vi "Grow Tail.vi"(8 "Keypress In":enum16{"Right", "Down", "Up", "Left"}(ring), 9 "Map In":u32[][](array[numeric]), 10 "Locations In":cluster{"Location Y":i32, "Location X":i32}[](array[cluster])=[{"Location Y"=12, "Location X"=8}, {"Location Y"=12, "Location X"=7}, {"Location Y"=12, "Location X"=6}, {"Location Y"=12, "Location X"=5}, {"Location Y"=12, "Location X"=4}]) -> (1 "Keypress Out":enum16{"Right", "Down", "Up", "Left"}(ring), 2 "Map Out":u32[][](array[numeric]), 3 "Locations Out":cluster{"Location Y":i32, "Location X":i32}[](array[cluster]))   [LabVIEW 2014]
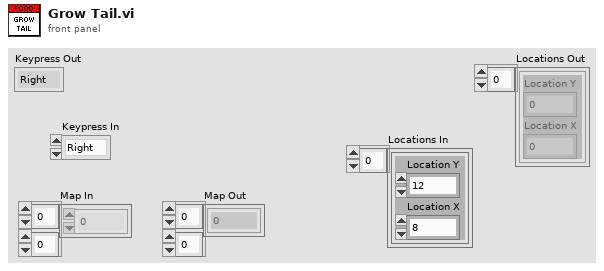
[diagram p1: front panel]
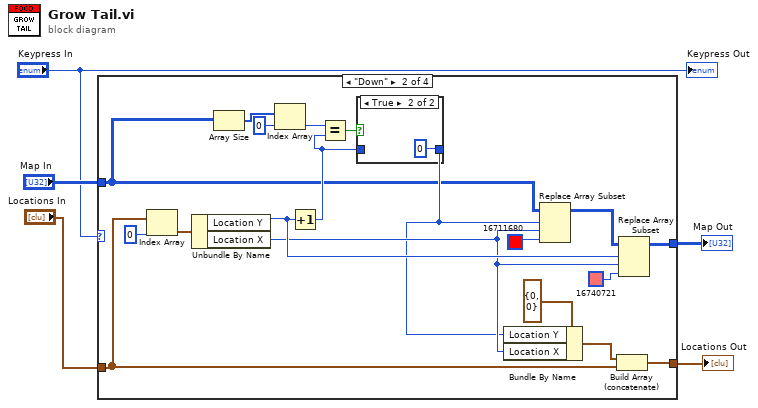
[diagram p0: block diagram]
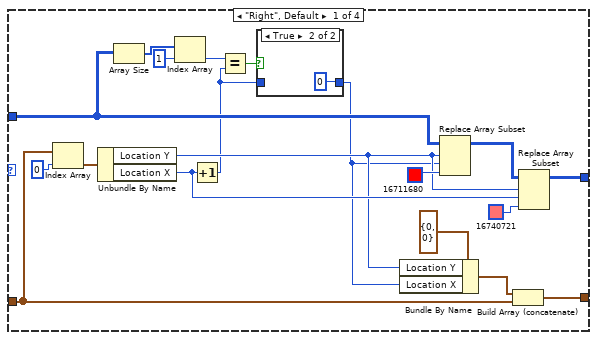
[diagram p2: hidden frame]
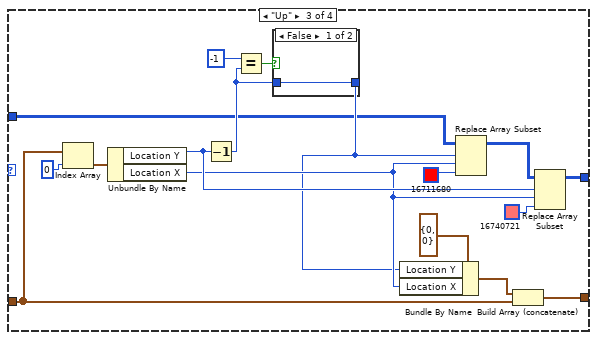
[diagram p5: hidden frame]
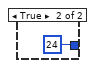
[diagram p6: hidden frame]
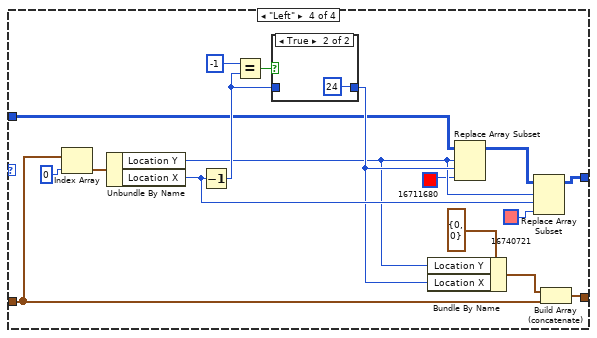
[diagram p7: hidden frame]
diagram:
  n1 = case shown="\"Down\"" "Keypress In" {
    tunnel: [w16 w28 w48 w68] -> w5
    tunnel: "Map In" -> [w13 w30 w51 w69]
    tunnel: [w7 w27 w49 w67] -> w3
    tunnel: "Locations In" -> [w6 w29 w50 w70]
    frame "Right", Default {
      n2 = Index Array(array=w6, index=0) -> (element=w23:cluster{"Location Y":i32, "Location X":i32})
      n3 = Unbundle By Name(w23) -> ("Location Y"=w15:i32, "Location X"=w19:i32)
      n4 = Array Size(array=w13) -> (size(s)=w12:i32[])
      n5 = Index Array(array=w12, index=1) -> (element=w10:i32)
      n6 = Increment(x=w19) -> (x+1=w9:i32)
      n7 = Equal?(x=w10, y=w9) -> (x = y?=w14:bool)
      n8 = case shown="True" w14 {
        tunnel: w9 -> [w25 _]
        tunnel: [w25 0] -> w8
        frame False {
        }
        frame True {
        }
      }
      n9 = Bundle By Name(cluster=cluster{"Location Y":i32, "Location X":i32} {"Location Y"=0, "Location X"=0} ("deleted portion"), "Location Y"=w15, "Location X"=w8) -> (w17:cluster{"Location Y":i32, "Location X":i32})
      n10 = Replace Array Subset(array=w13, new element=u32 16711680, index (row)=w15, index (col)=w8) -> (w21:u32[][])
      n11 = Build Array (concatenate)(w17, w6) -> (w16:cluster{"Location Y":i32, "Location X":i32}[])
      n12 = Replace Array Subset(array=w21, new element=u32 16740721, index (row)=w15, index (col)=w19) -> (w7:u32[][])
    }
    frame "Down" {
      n13 = Index Array(array=w29, index=0) -> (element=w32:cluster{"Location Y":i32, "Location X":i32})
      n14 = Unbundle By Name(w32) -> ("Location Y"=w45:i32, "Location X"=w43:i32)
      n15 = Array Size(array=w30) -> (size(s)=w38:i32[])
      n16 = Index Array(array=w38, index=0) -> (element=w40:i32)
      n17 = Increment(x=w45) -> (x+1=w41:i32)
      n18 = Equal?(x=w40, y=w41) -> (x = y?=w37:bool)
      n19 = case shown="True" w37 {
        tunnel: w41 -> [w46 _]
        tunnel: [w46 0] -> w42
        frame False {
        }
        frame True {
        }
      }
      n20 = Bundle By Name(cluster=cluster{"Location Y":i32, "Location X":i32} {"Location Y"=0, "Location X"=0} ("deleted portion"), "Location Y"=w42, "Location X"=w43) -> (w36:cluster{"Location Y":i32, "Location X":i32})
      n21 = Replace Array Subset(array=w30, new element=u32 16711680, index (row)=w42, index (col)=w43) -> (w33:u32[][])
      n22 = Build Array (concatenate)(w36, w29) -> (w28:cluster{"Location Y":i32, "Location X":i32}[])
      n23 = Replace Array Subset(array=w33, new element=u32 16740721, index (row)=w45, index (col)=w43) -> (w27:u32[][])
    }
    frame "Up" {
      n24 = Index Array(array=w50, index=0) -> (element=w53:cluster{"Location Y":i32, "Location X":i32})
      n25 = Unbundle By Name(w53) -> ("Location Y"=w62:i32, "Location X"=w60:i32)
      n26 = Decrement(x=w62) -> (x-1=w63:i32)
      n27 = Equal?(x=-1, y=w63) -> (x = y?=w58:bool)
      n28 = case shown="False" w58 {
        tunnel: w63 -> [w65 _]
        tunnel: [w65 24] -> w59
        frame False {
        }
        frame True {
        }
      }
      n29 = Bundle By Name(cluster=cluster{"Location Y":i32, "Location X":i32} {"Location Y"=0, "Location X"=0} ("deleted portion"), "Location Y"=w59, "Location X"=w60) -> (w57:cluster{"Location Y":i32, "Location X":i32})
      n30 = Replace Array Subset(array=w51, new element=u32 16711680, index (row)=w59, index (col)=w60) -> (w54:u32[][])
      n31 = Build Array (concatenate)(w57, w50) -> (w48:cluster{"Location Y":i32, "Location X":i32}[])
      n32 = Replace Array Subset(array=w54, new element=u32 16740721, index (row)=w62, index (col)=w60) -> (w49:u32[][])
    }
    frame "Left" {
      n33 = Index Array(array=w70, index=0) -> (element=w72:cluster{"Location Y":i32, "Location X":i32})
      n34 = Unbundle By Name(w72) -> ("Location Y"=w78:i32, "Location X"=w81:i32)
      n35 = Decrement(x=w81) -> (x-1=w82:i32)
      n36 = Equal?(x=-1, y=w82) -> (x = y?=w79:bool)
      n37 = case shown="True" w79 {
        tunnel: w82 -> [w84 _]
        tunnel: [w84 24] -> w80
        frame False {
        }
        frame True {
        }
      }
      n38 = Bundle By Name(cluster=cluster{"Location Y":i32, "Location X":i32} {"Location Y"=0, "Location X"=0} ("deleted portion"), "Location Y"=w78, "Location X"=w80) -> (w77:cluster{"Location Y":i32, "Location X":i32})
      n39 = Replace Array Subset(array=w69, new element=u32 16711680, index (row)=w78, index (col)=w80) -> (w74:u32[][])
      n40 = Replace Array Subset(array=w74, new element=u32 16740721, index (row)=w78, index (col)=w81) -> (w67:u32[][])
      n41 = Build Array (concatenate)(w77, w70) -> (w68:cluster{"Location Y":i32, "Location X":i32}[])
    }
  }
  "Map Out" <- w3
  "Locations Out" <- w5
  "Keypress Out" <- "Keypress In"
